vi "Color_Sensor_Logic.vi"() -> ()   [LabVIEW 2020]
uses:
  <vilib>/Rock Robotics/Network Tables/NT Write String.vi
  <vilib>/Rock Robotics/Network Tables/NT Read String.vi
panel:
  in  "Red/Blue":u32(colorbox)
  out "B":u8
  out "G":u8
  out "R":u8
  out "Color":u32(colorbox)
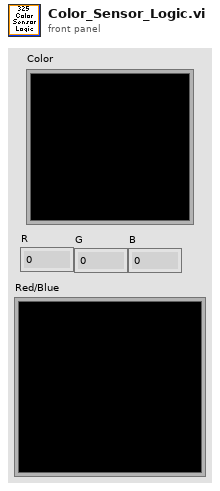
[diagram p1: front panel]
types:
  T1 = typedef "Color Sensor V3 DevRef.ctl" = cluster{"I2CDevRef":T2}
  T2 = typedef "WPI_I2CDevRef.ctl" = cluster{"DevStatus":errorcluster, "Device Address":u8, "Handle":i32, "I2C Bus":T3}
  T3 = typedef "i2c_bus.ctl" = enum16{"I2C On-Board", "I2C MXP", "Invalid"}
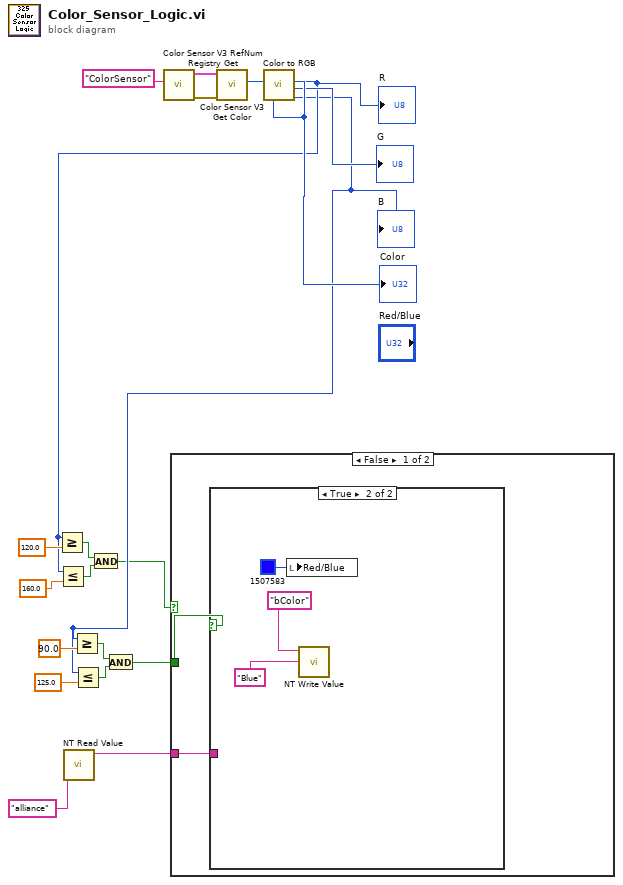
[diagram p0: block diagram]
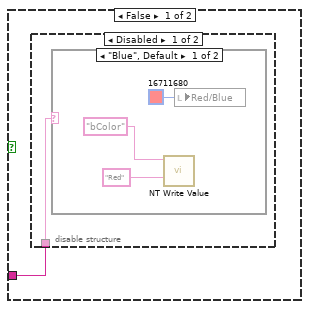
[diagram p2: hidden frame]
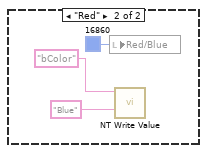
[diagram p3: hidden frame]
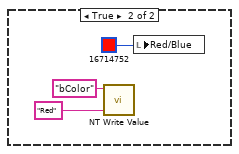
[diagram p5: hidden frame]
diagram:
  n1 = call-poly <vilib>:"NT Read Value.vi"("Name"="alliance") -> ("String"=w1:string)  [unwired: 9 in, 1 out]
  n2 = call <vilib>:"Color Sensor V3 RefNum Registry Get.vi"("refnum name"="ColorSensor") -> ("error out"=w17:errorcluster, "ColorSensorDevRef"=w18:T1)  [unwired: 9 in]
  n3 = call <vilib>:"Color Sensor V3 Get Color.vi"("error in (no error)"=w17, "ColorSensorDevRef"=w18) -> ("Color"=w16:u32)  [unwired: 6 in, 3 out]
  "Color" <- w16
  n4 = call <vilib>:"Color to RGB.vi"("Color"=w16) -> ("R"=w10:u8, "G"=→"G":u8, "B"=w5:u8)  [unwired: 1 out]
  "R" <- w10
  "B" <- w5
  n5 = Greater Or Equal?(x=w10, y=120.0) -> (x >= y?=w13:bool)
  n6 = Less Or Equal?(x=w10, y=160.0) -> (x <= y?=w14:bool)
  n7 = Greater Or Equal?(x=w5, y=90.0) -> (x >= y?=w8:bool)
  n8 = Less Or Equal?(x=w5, y=125.0) -> (x <= y?=w9:bool)
  n9 = And(x=w13, y=w14) -> (x .and. y?=w4:bool)
  n10 = And(x=w8, y=w9) -> (x .and. y?=w3:bool)
  n11 = case shown="False" w4 {
    tunnel: w3 -> [w21 _]
    tunnel: w1 -> [w20 _]
    frame False {
      n12 = case shown="True" w21 {
        tunnel: w20 -> [w22 _]
        frame False {
          n13 = disable-structure shown="Disabled" {
            disable-tunnel: w22 -> [w23 _]
            frame Disabled {
              n14 = case shown="\"Blue\", Default" w23 {
                frame "Blue", Default {
                  n15 = call-poly <vilib>:"NT Write Value.vi"("String"="Red", "Name"="bColor") -> ()  [unwired: 9 in, 1 out]
                  n16 = local write "Red/Blue"(u32 16711680 ("Color Box")) -> ()
                }
                frame "Red" {
                  n17 = local write "Red/Blue"(u32 16860 ("Red/Blue")) -> ()
                  n18 = call-poly <vilib>:"NT Write Value.vi"("String"="Blue", "Name"="bColor") -> ()  [unwired: 9 in, 1 out]
                }
              }
            }
            frame Enabled {
            }
          }
        }
        frame True {
          n19 = local write "Red/Blue"(u32 1507583 ("Color Box")) -> ()
          n20 = call-poly <vilib>:"NT Write Value.vi"("String"="Blue", "Name"="bColor") -> ()  [unwired: 9 in, 1 out]
        }
      }
    }
    frame True {
      n21 = call-poly <vilib>:"NT Write Value.vi"("String"="Red", "Name"="bColor") -> ()  [unwired: 9 in, 1 out]
      n22 = local write "Red/Blue"(u32 16714752) -> ()
    }
  }
